vi "to_xml.vi"(8 "error in":errorcluster, 11 "DAQmx Pulse Settings":T1={"Enable DAQmx Pulses"=FALSE, "DAQmx Physical Channels"="Dev2/port0_32", "Clock Rate"=10000000.0, "units/sec (ms=1000)"=1000.0, "Start Trigger"={"Wait for start trigger?"=FALSE, "source"="/Dev1/PFI0", "edge"=10280}, "Timing Sequence Control"=[["camera/repump", "1", "0", "", "", "", "", "", "", "", "", "", "", "", "", "", "", "", "", "", "1000", "1000", "1000", "1000", "", "", "", "", "", "", "", "", "", "", "", "", "", "", ""], ["probe", "1", "0", "", "", "", "", "", "", "", "", "", "", "", "", "", "", "", "", "", "", "", "", "", "", "", "", "", "", "", "", "", "", "", "", "", "", "", ""], ["bias field", "1", "0", "", "", "", "", "", "", "", "", "", "", "", "", "", "", "", "", "", "", "", "", "", "", "", "", "", "", "", "", "", "", "", "", "", "", "", ""], ["switch 1 MOT to PGC freq shift", "1", "0", "", "", "", "", "", "", "", "", "", "", "", "", "", "", "", "", "", "", "", "", "", "", "", "", "", "", "", "", "", "", "", "", "", "", "", ""], ["B field", "1", "0", "", "", "", "", "", "", "", "", "", "", "", "", "", "", "", "", "", "", "", "", "", "", "", "", "", "", "", "", "", "", "", "", "", "", "", ""], ["trigger PD1", "1", "0", "", "", "", "", "", "", "", "", "", "", "", "", "", "", "", "", "", "", "", "", "", "", "", "", "", "", "", "", "", "", "", "", "", "", "", ""], ["rf switch 2 cooling laser on/off", "1", "0", "", "", "", "", "", "", "", "", "", "", "", "", "", "", "", "", "", "", "", "", "", "", "", "", "", "", "", "", "", "", "", "", "", "", "", ""], ["Bob switch", "1", "0", "", "", "", "", "", "", "", "", "", "", "", "", "", "", "", "", "", "", "", "", "", "", "", "", "", "", "", "", "", "", "", "", "", "", "", ""], ["switch 3 894nm", "1", "0", "", "", "", "", "", "", "", "", "", "", "", "", "", "", "", "", "", "", "", "", "", "", "", "", "", "", "", "", "", "", "", "", "", "", "", ""], ["clock trigger", "1", "0", "", "", "", "", "", "", "", "", "", "", "", "", "", "", "", "", "", "", "", "", "", "", "", "", "", "", "", "", "", "", "", "", "", "", "", ""], ["Raman", "1", "0", "", "", "", "", "", "", "", "", "", "", "", "", "", "", "", "", "", "", "", "", "", "", "", "", "", "", "", "", "", "", "", "", "", "", "", ""], ["684 shutter", "1", "0", "", "", "", "", "", "", "", "", "", "", "", "", "", "", "", "", "", "", "", "", "", "", "", "", "", "", "", "", "", "", "", "", "", "", "", ""], ["repumper switch 2", "1", "0", "", "", "", "", "", "", "", "", "", "", "", "", "", "", "", "", "", "", "", "", "", "", "", "", "", "", "", "", "", "", "", "", "", "", "", ""], ["further PGC", "1", "0", "", "", "", "", "", "", "", "", "", "", "", "", "", "", "", "", "", "", "", "", "", "", "", "", "", "", "", "", "", "", "", "", "", "", "", ""], ["pumping laser switch 2", "1", "0", "", "", "", "", "", "", "", "", "", "", "", "", "", "", "", "", "", "", "", "", "", "", "", "", "", "", "", "", "", "", "", "", "", "", "", ""], ["Raman 2", "1", "0", "", "", "", "", "", "", "", "", "", "", "", "", "", "", "", "", "", "", "", "", "", "", "", "", "", "", "", "", "", "", "", "", "", "", "", ""], ["MOT beam on/off switch 2", "1", "0", "", "", "", "", "", "", "", "", "", "", "", "", "", "", "", "", "", "", "", "", "", "", "", "", "", "", "", "", "", "", "", "", "", "", "", ""], ["push beam switch 2", "1", "0", "", "", "", "", "", "", "", "", "", "", "", "", "", "", "", "", "", "", "", "", "", "", "", "", "", "", "", "", "", "", "", "", "", "", "", ""], ["532 AOM", "1", "0", "", "", "", "", "", "", "", "", "", "", "", "", "", "", "", "", "", "", "", "", "", "", "", "", "", "", "", "", "", "", "", "", "", "", "", ""], ["Andor Luca Trigger", "1", "0", "", "", "", "", "", "", "", "", "", "", "", "", "", "", "", "", "", "", "", "", "", "", "", "", "", "", "", "", "", "", "", "", "", "", "", ""], ["trigger PD2", "1", "0", "", "", "", "", "", "", "", "", "", "", "", "", "", "", "", "", "", "", "", "", "", "", "", "", "", "", "", "", "", "", "", "", "", "", "", ""], ["1038 switch", "1", "0", "", "", "", "", "", "", "", "", "", "", "", "", "", "", "", "", "", "", "", "", "", "", "", "", "", "", "", "", "", "", "", "", "", "", "", ""], ["459 switch", "1", "0", "", "", "", "", "", "", "", "", "", "", "", "", "", "", "", "", "", "", "", "", "", "", "", "", "", "", "", "", "", "", "", "", "", "", "", ""], ["", "", "", "", "", "", "", "", "", "", "", "", "", "", "", "", "", "", "", "", "", "", "", "", "", "", "", "", "", "", "", "", "", "", "", "", "", "", ""], ["", "", "", "", "", "", "", "", "", "", "", "", "", "", "", "", "", "", "", "", "", "", "", "", "", "", "", "", "", "", "", "", "", "", "", "", "", "", ""], ["", "", "", "", "", "", "", "", "", "", "", "", "", "", "", "", "", "", "", "", "", "", "", "", "", "", "", "", "", "", "", "", "", "", "", "", "", "", ""], ["", "", "", "", "", "", "", "", "", "", "", "", "", "", "", "", "", "", "", "", "", "", "", "", "", "", "", "", "", "", "", "", "", "", "", "", "", "", ""], ["", "", "", "", "", "", "", "", "", "", "", "", "", "", "", "", "", "", "", "", "", "", "", "", "", "", "", "", "", "", "", "", "", "", "", "", "", "", ""], ["", "", "", "", "", "", "", "", "", "", "", "", "", "", "", "", "", "", "", "", "", "", "", "", "", "", "", "", "", "", "", "", "", "", "", "", "", "", ""], ["", "", "", "", "", "", "", "", "", "", "", "", "", "", "", "", "", "", "", "", "", "", "", "", "", "", "", "", "", "", "", "", "", "", "", "", "", "", ""], ["", "", "", "", "", "", "", "", "", "", "", "", "", "", "", "", "", "", "", "", "", "", "", "", "", "", "", "", "", "", "", "", "", "", "", "", "", "", ""], ["", "", "", "", "", "", "", "", "", "", "", "", "", "", "", "", "", "", "", "", "0", "", "", "", "", "", "", "", "", "", "", "", "", "", "", "", "", "", ""]]} {"Start Trigger"."edge" items=["Rising"=10280, "Falling"=10171]; "Clock Rate" min=0.0 max=200000000.0 format="%.2p"}) -> (0 "error out":errorcluster, 3 "DAQmx settings string":string)   [LabVIEW 2013, in "DAQmx_pulse_out.lvclass"]
doc: "Saves DAQmx pulse output settings to xml in the format:\n\n<EnableDAQmxPulses>%b</EnableDAQmxPulses>\n<ResourceName>%s</ResourceName>\n<ClockRate>%f</ClockRate>\n<unitsPerSecond>%f</unitsPerSecond>\n<StartTrigger.WaitForStartTrigger>%b</StartTrigger.WaitForStartTrigger>\n<StartTrigger.source>%s</StartTrigger.source>\n<StartTrigger.edge>%s</StartTrigger.edge>\n<TimingSequenceControl columns=\"Description, Active?, Idle State,Off 0,On 0,Off 1,On 1,etc.\">\n<channel>%s</channel>\n</TimingSequenceControl>\n\nMTL 2013 Jan 1"
uses:
  DAQmx_pulse_out.lvclass
  settings.ctl
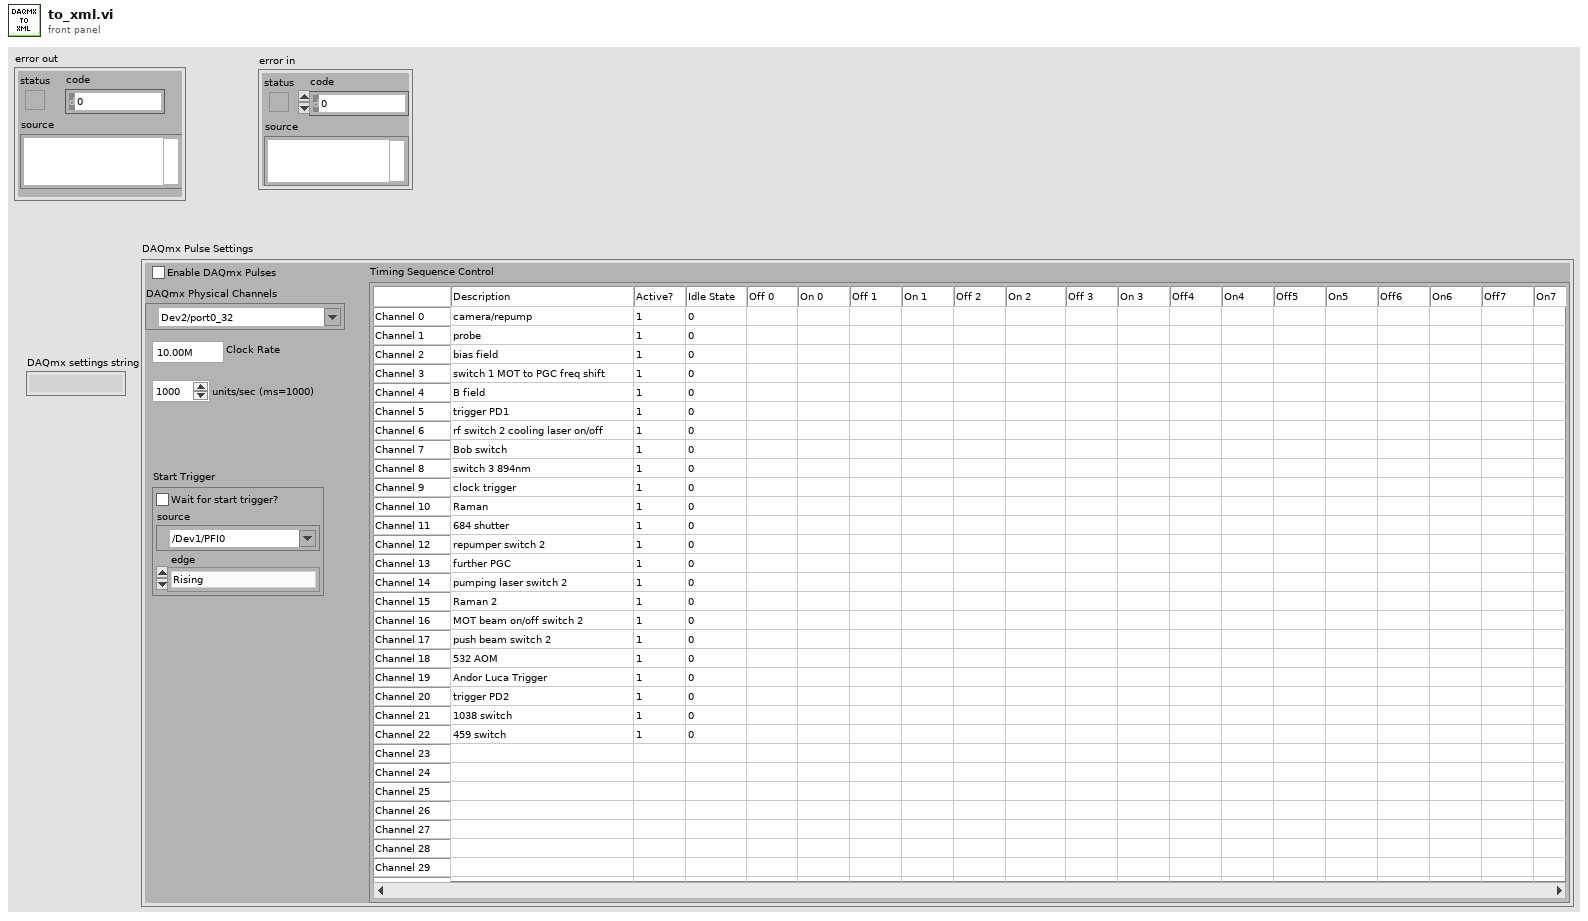
[diagram p1: front panel]
types:
  T1 = typedef "DAQmx_pulse_out.lvclass/settings.ctl" = cluster{"Enable DAQmx Pulses":bool, "DAQmx Physical Channels":tag, "Clock Rate":dbl, "units/sec (ms=1000)":dbl, "Start Trigger":cluster{"Wait for start trigger?":bool, "source":tag, "edge":i32}, "Timing Sequence Control":string[][]}
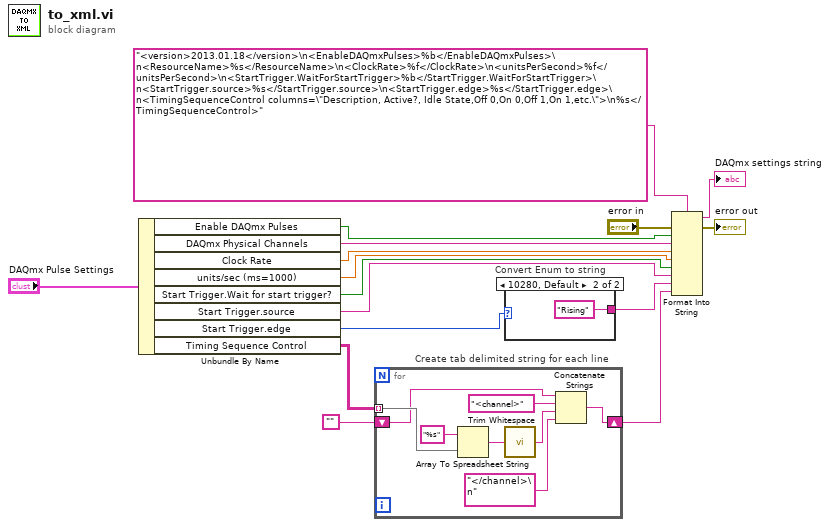
[diagram p0: block diagram]
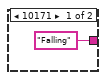
[diagram p2: hidden frame]
diagram:
  n1 = Unbundle By Name("DAQmx Pulse Settings") -> ("Enable DAQmx Pulses"=w12:bool, "DAQmx Physical Channels"=w11:tag, "Clock Rate"=w10:dbl, "units/sec (ms=1000)"=w9:dbl, "Start Trigger.Wait for start trigger?"=w8:bool, "Start Trigger.source"=w7:tag, "Start Trigger.edge"=w6:i32, "Timing Sequence Control"=w4:string[][])
  n2 = for "Create tab delimited string for each line" {
    tunnel: w4 -> [w24] mode=indexing
    shift-right: [w20] -> w1
    shift-left: "" -> [w19]
    n3 = Array To Spreadsheet String(array=w24, 3:"%s" ("format string")) -> (spreadsheet string=w18:string)  [unwired: 1 in]
    n4 = call <vilib>:"Trim Whitespace.vi"("string"=w18) -> ("trimmed string"=w17:string)  [unwired: 1 in]
    n5 = Concatenate Strings(w19, "<channel>" ("string"), w17, "</channel>\n" ("string")) -> (w20:string)
  }
  n6 = case "Convert Enum to string" shown="10280, Default" w6 {
    tunnel: ["Falling" "Rising"] -> w5
    frame 10171 {
    }
    frame 10280, Default {
    }
  }
  n7 = Format Into String(format string="<version>2013.01.18</version>\n<EnableDAQmxPulses>%b</EnableDAQmxPulses>\n<ResourceName>%s</ResourceName>\n<ClockRate>%f</ClockRate>\n<unitsPerSecond>%f</unitsPerSecond>\n<StartTrigger.WaitForStartTrigger>%b</StartTrigger.WaitForStartTrigger>\n<StartTrigger.source>%s</StartTrigger.source>\n<StartTrigger.edge>%s</StartTrigger.edge>\n<TimingSequenceControl columns=\"Description, Active?, Idle State,Off 0,On 0,Off 1,On 1,etc.\">\n%s</TimingSequenceControl>", error in="error in", w12, w11, w10, w9, w8, w7, w5, w1) -> (resulting string=→"DAQmx settings string":string, error out=→"error out":errorcluster)  [unwired: 1 in]
